vi "startUp.vi"(8 "error in (no error)":errorcluster, 10 "ScriptEvent":refnum<class "ScriptEvent.lvclass">, 11 "RampAction in":refnum<class "RampAction.lvclass">) -> (0 "error out":errorcluster, 3 "RampAction out":refnum<class "RampAction.lvclass">)   [LabVIEW 2009, in "Views.lvlib" / "ScriptEditor.lvlib" / "RampAction.lvclass"]
uses:
  RampAction.lvclass
  Tools/Scripting/ScriptingEvent/ScriptEvent.lvclass
  Tools/Scripting/ScriptingEvent/ScriptEvents/Ramp/RampEvent/RampEvent.lvclass
  RampAction.lvclass/RampAction.ctl
  ActionPanel.lvclass
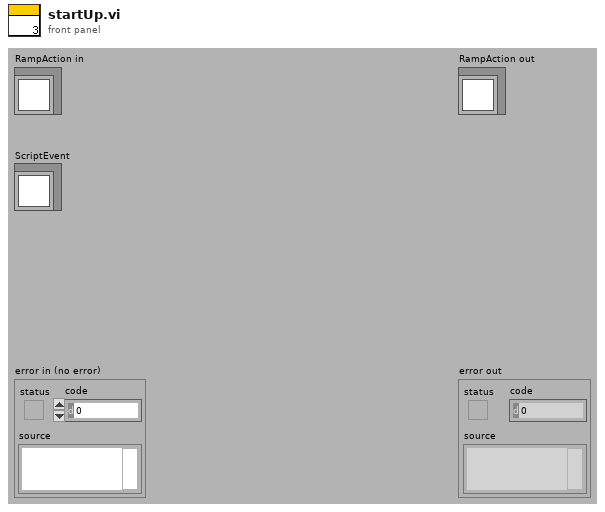
[diagram p1: front panel]
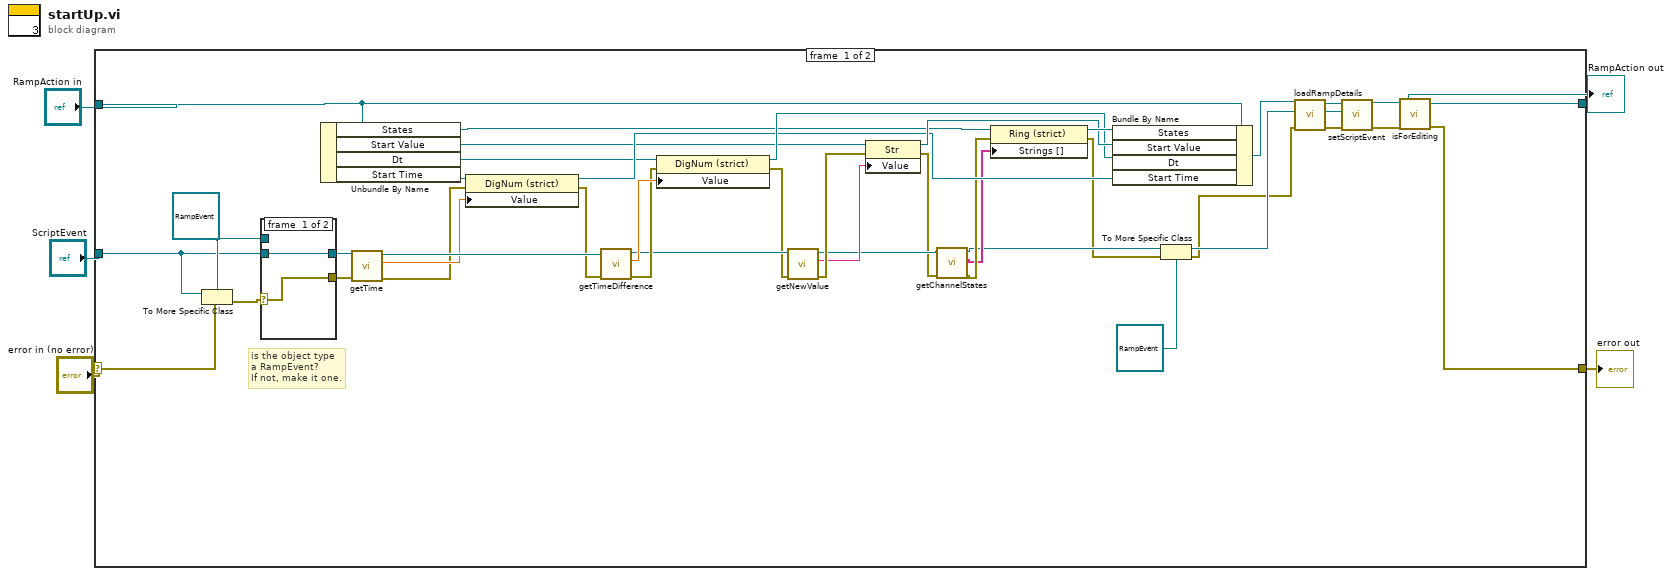
[diagram p0: block diagram]
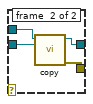
[diagram p2: hidden frame]
diagram:
  n1 = case shown="No Error" "error in (no error)" {
    selector: "error in (no error)" -> [w21 w54]
    tunnel: "RampAction in" -> [w33 w55]
    tunnel: "ScriptEvent" -> [w15 _]
    tunnel: [w6 w55] -> w2
    tunnel: [w7 w54] -> w1
    frame #0 {
      w23 = refnum<class "RampEvent.lvclass"> refnum ("RampEvent in")
      # "is the object type\na RampEvent?\nIf not, make it one."
      n2 = To More Specific Class(target class=w23, reference=w15, error in=w21) -> (error out=w24:errorcluster)  [unwired: 1 out]
      n3 = case shown="Error" w24 {
        selector: w24 -> [w48 _]
        tunnel: w15 -> [w49 w52]
        tunnel: w23 -> [_ w53]
        tunnel: [w48 w51] -> w22
        tunnel: [w49 w50] -> w20
        frame #0 {
        }
        frame #1 {
          n4 = call-dynamic "copy.vi"("ScriptEventForCopy"=w52, "RampEvent in"=w53) -> ("error out"=w51:errorcluster, "RampEvent Copy"=w50:refnum<class "RampEvent.lvclass">)  [unwired: 8 in]
        }
      }
      n5 = Unbundle By Name(w33) -> ("States"=w27:refnum<vi>, "Start Value"=w28:refnum<vi>, "Dt"=w26:refnum<vi>, "Start Time"=w25:refnum<vi>)
      n6 = call "getTime.vi"("error in (no error)"=w22, "ScriptEvent.lvclass in"=w20) -> ("error out"=w45:errorcluster, "time"=w46:dbl, "ScriptEvent.lvclass out"=w47:refnum<class "ScriptEvent.lvclass">)  [unwired: 7 in]
      n7 = property class="DigNum (strict)"(reference=w25, error in=w45, "Value"=w46) -> (reference out=w34:refnum<vi>, error out=w44:errorcluster)
      n8 = call "getTimeDifference.vi"("error in (no error)"=w44, "ScriptEvent.lvclass in"=w47) -> ("error out"=w42:errorcluster, "time difference"=w43:dbl, "ScriptEvent.lvclass out"=w41:refnum<class "ScriptEvent.lvclass">)  [unwired: 7 in]
      n9 = property class="DigNum (strict)"(reference=w26, error in=w42, "Value"=w43) -> (reference out=w35:refnum<vi>, error out=w40:errorcluster)
      n10 = call "getNewValue.vi"("error in (no error)"=w40, "ScriptEvent.lvclass in"=w41) -> ("error out"=w39:errorcluster, "newValue"=w38:string, "ScriptEvent.lvclass out"=w32:refnum<class "ScriptEvent.lvclass">)  [unwired: 7 in]
      n11 = property class="Str"(reference=w28, error in=w39, "Value"=w38) -> (reference out=w36:refnum<vi>, error out=w31:errorcluster)
      n12 = call-dynamic "getChannelStates.vi"("error in (no error)"=w31, "ScriptEvent in"=w32) -> ("error out"=w30:errorcluster, "statesValues"=w29:string[], "ScriptEvent out"=w14:refnum<class "ScriptEvent.lvclass">)  [unwired: 7 in]
      n13 = property class="Ring (strict)"(reference=w27, error in=w30, "Strings []"=w29) -> (reference out=w37:refnum<vi>, error out=w11:errorcluster)
      n14 = Bundle By Name(cluster=w33, "States"=w37, "Start Value"=w36, "Dt"=w35, "Start Time"=w34) -> (w19:refnum<class "RampAction.lvclass">)
      n15 = To More Specific Class(target class=refnum<class "RampEvent.lvclass"> refnum ("RampEvent in"), reference=w14, error in=w11) -> (specific class reference=w12:refnum<class "RampEvent.lvclass">, error out=w10:errorcluster)
      n16 = call "loadRampDetails.vi"("error in (no error)"=w10, "RampEvent in"=w12, "RampAction in"=w19) -> ("error out"=w16:errorcluster, "RampEvent out"=w17:refnum<class "RampEvent.lvclass">, "RampAction out"=w18:refnum<class "RampAction.lvclass">)  [unwired: 6 in]
      n17 = call "setScriptEvent.vi"("error in (no error)"=w16, "ScriptEvent.lvclass"=w17, "ActionPanel.lvclass in"=w18) -> ("error out"=w9:errorcluster, "ActionPanel.lvclass out"=w8:refnum<class "RampAction.lvclass">)  [unwired: 7 in]
      n18 = call-dynamic "isForEditing.vi"("error in (no error)"=w9, "RampAction in"=w8) -> ("error out"=w7:errorcluster, "RampAction out"=w6:refnum<class "RampAction.lvclass">)  [unwired: 7 in, 1 out]
    }
    frame #1 {
    }
  }
  "error out" <- w1
  "RampAction out" <- w2
